vi "Add Result.vi"(8 "error in (no error)":errorcluster, 9 "Sequenc Context":refnum<class "Configuration.lvclass">, 10 "TestStand Result":T1, 11 "TestStand Result Handler In":refnum<class "TestStand Result Handler.lvclass">) -> (0 "error out":errorcluster, 3 "TestStand Result Handler Out":refnum<class "TestStand Result Handler.lvclass">)   [LabVIEW 2020, in "Astemes_CSVReportPlugin.lvlib" / "TestStand Result Handler.lvclass"]
uses:
  TestStand Result Handler.lvclass
  TestStand Result.ctl
  Configuration/Configuration.lvclass
  TestStand Result Handler.lvclass/TestStand Result Handler.ctl
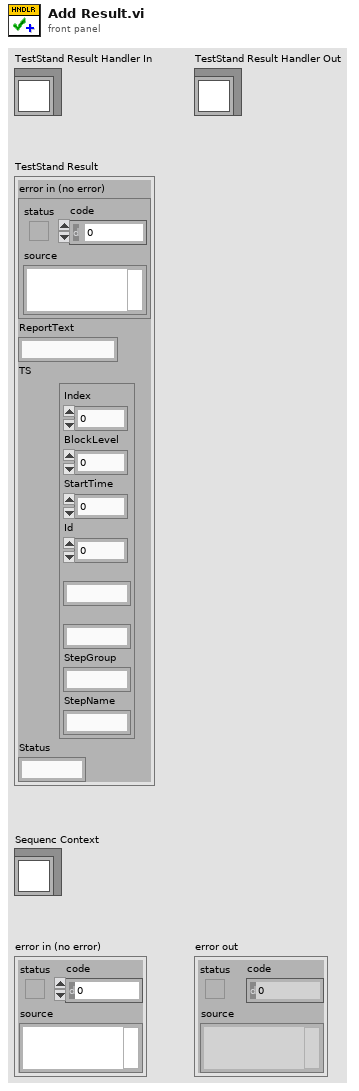
[diagram p1: front panel]
types:
  T1 = typedef "Astemes_CSVReportPlugin.lvlib/TestStand Result Handler.lvclass/TestStand Result.ctl" = cluster{"error in (no error)":errorcluster, "ReportText":string, "TS":cluster{"Index":i32, "BlockLevel":i32, "StartTime":dbl, "Id":i32, "StepType":string, "StepID":string, "StepGroup":string, "StepName":string}, "Status":string}
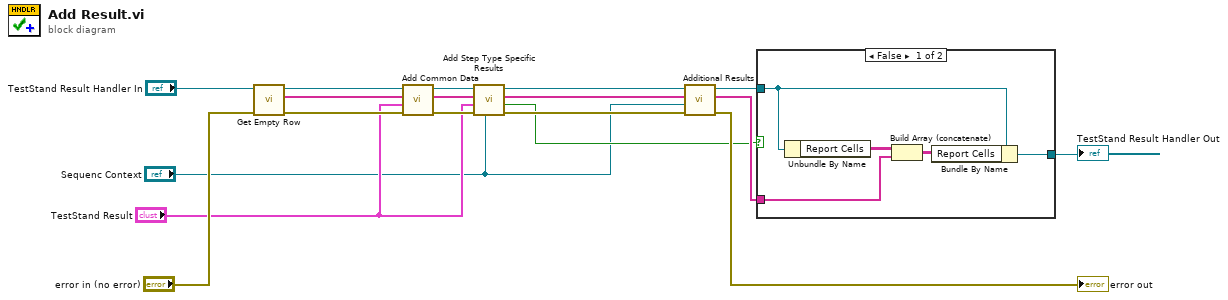
[diagram p0: block diagram]
diagram:
  n1 = call "Get Empty Row.vi"("error in (no error)"="error in (no error)", "Result Handler"="TestStand Result Handler In") -> ("error out"=w16:errorcluster, "Empty Row"=w10:string[], "Result Handler"=w9:refnum<class "TestStand Result Handler.lvclass">)  [unwired: 7 in]
  n2 = call "Add Common Data.vi"("error in (no error)"=w16, "TestStand Result"="TestStand Result", "Empty Row"=w10, "Result Handler"=w9) -> ("error out"=w14:errorcluster, "Array"=w1:string[], "Result Handler 2"=w4:refnum<class "TestStand Result Handler.lvclass">)  [unwired: 5 in]
  n3 = call "Add Step Type Specific Results.vi"("Configuration in"="Sequenc Context", "error in (no error)"=w14, "TestStand Result"="TestStand Result", "Array in"=w1, "Result Handler"=w4) -> ("error out"=w18:errorcluster, "Ignore?"=w8:bool, "Array out"=w7:string[], "Result Handler Out"=w2:refnum<class "TestStand Result Handler.lvclass">)  [unwired: 3 in]
  n4 = call-dynamic "Additional Results.vi"("error in (no error)"=w18, "Sequenc Context"="Sequenc Context", "Array in"=w7, "TestStand Result Handler in"=w2) -> ("error out"=→"error out":errorcluster, "Array"=w11:string[], "TestStand Result Handler out"=w13:refnum<class "TestStand Result Handler.lvclass">)  [unwired: 5 in]
  n5 = case shown="False" w8 {
    tunnel: [w21 w24] -> w17
    tunnel: w13 -> [w20 w24]
    tunnel: w11 -> [w19 _]
    frame False {
      n6 = Unbundle By Name(w20) -> ("Report Cells"=w22:string[][])
      n7 = Build Array (concatenate)(w22, w19) -> (w23:string[][])
      n8 = Bundle By Name(cluster=w20, "Report Cells"=w23) -> (w21:refnum<class "TestStand Result Handler.lvclass">)
    }
    frame True {
    }
  }
  "TestStand Result Handler Out" <- w17
